vi "Close Session.vi"(8 "error in (no error)":errorcluster, 11 "MB session in":refnum<class "MB_Master.lvclass">) -> (0 "error out":errorcluster)   [LabVIEW 2016, in "MB Master.lvlib" / "MB_Master.lvclass"]
doc: "Close the Modbus session. This will release the mutex and close the serial port."
uses:
  MB_Master.lvclass
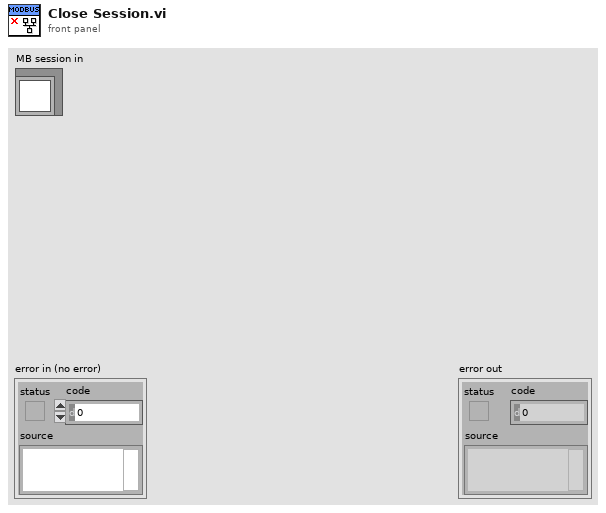
[diagram p1: front panel]
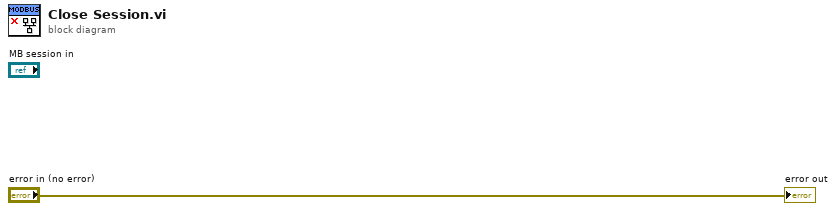
[diagram p0: block diagram]
diagram:
  "error out" <- "error in (no error)"
